vi "Broadcast.vi"(8 "error in (no error)":errorcluster, 10 "Brower Controller_Q":refnum<class "Message Enqueuer.lvclass">, 11 "GUI Control Builder Director in":refnum<class "GUI Control Builder Director.lvclass">) -> (0 "error out":errorcluster, 3 "GUI Control Builder Director out":refnum<class "GUI Control Builder Director.lvclass">)   [LabVIEW 2015, in "GUI Control Builder Director.lvclass"]
uses:
  GUI Control Builder Director.lvclass
  <vilib>/ActorFramework/Message Enqueuer/Message Enqueuer.lvclass
  GUI Control Builder Director.lvclass/GUI Control Builder Director.ctl
  Control Builders/GUI Control Builder/GUI Control Builder.lvclass
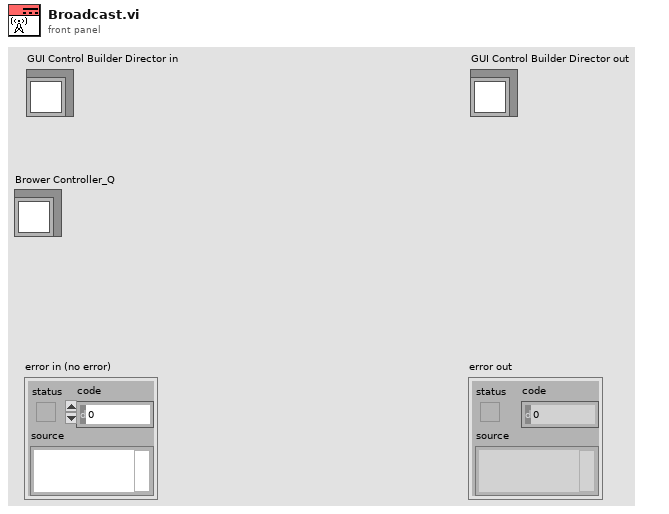
[diagram p1: front panel]
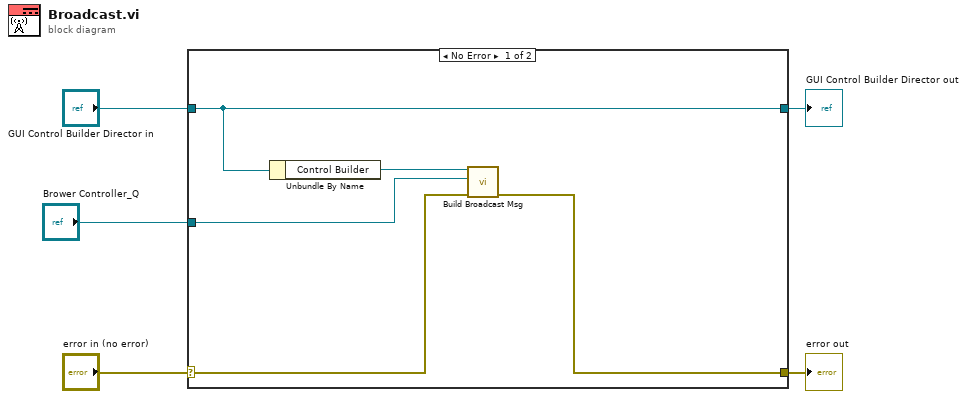
[diagram p0: block diagram]
diagram:
  n1 = case shown="No Error" "error in (no error)" {
    selector: "error in (no error)" -> [w7 w12]
    tunnel: [w6 w12] -> w4
    tunnel: [w10 w11] -> w2
    tunnel: "GUI Control Builder Director in" -> [w10 w11]
    tunnel: "Brower Controller_Q" -> [w8 _]
    frame No Error {
      n2 = Unbundle By Name(w10) -> ("Control Builder"=w9:refnum<class "GUI Control Builder.lvclass">)
      n3 = call-dynamic "Build Broadcast Msg.vi"("error in (no error)"=w7, "Brower Controller_Q"=w8, "Control Builder in"=w9) -> ("error out"=w6:errorcluster)  [unwired: 7 in, 1 out]
    }
    frame Error {
    }
  }
  "error out" <- w4
  "GUI Control Builder Director out" <- w2
